vi "Mouse Left Click at Set Position.vi"(1 "Click position file path":path) -> (0 "Error out":errorcluster)   [LabVIEW 2015]
panel:
  out "Y":i32
  out "X":i32
  # "PN 18/11/2015"
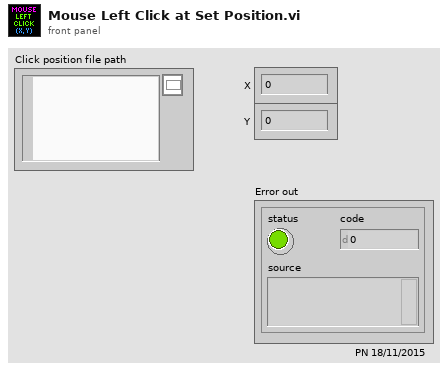
[diagram p1: front panel]
types:
  T1 = enum16{"open", "replace", "create", "open or create", "replace or create", "replace or create with confirmation"}
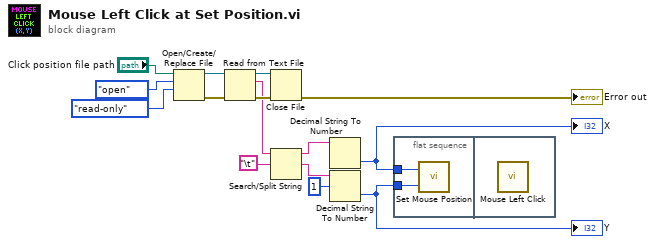
[diagram p0: block diagram]
diagram:
  n1 = Open/Create/Replace File(file path (use dialog)="Click position file path", operation (0:open)=T1."open", access (0:read/write)=enum16{"read/write", "read-only", "write-only"}."read-only") -> (refnum out=w14:refnum<file>, error out=w15:errorcluster)  [unwired: 3 in, 1 out]
  n2 = Read from Text File(file (use dialog)=w14, error in=w15) -> (refnum out=w10:refnum<file>, text=w4:string, error out=w9:errorcluster)  [unwired: 2 in, 1 out]
  n3 = Close File(refnum=w10, error in=w9) -> (error out=→"Error out":errorcluster)  [unwired: 1 out]
  n4 = Search/Split String(string=w4, search string/char (-)="\t") -> (substring before match=w2:string, match + rest of string=w1:string)  [unwired: 1 in, 1 out]
  n5 = Decimal String To Number(string=w2) -> (number=w7:i32)  [unwired: 2 in, 1 out]
  "X" <- w7
  n6 = Decimal String To Number(string=w1, offset=1) -> (number=w6:i32)  [unwired: 1 in, 1 out]
  "Y" <- w6
  n7 = flat-sequence {
    tunnel: w7 -> [w17]
    tunnel: w6 -> [w16]
    frame #0 {
      n8 = call "Set Mouse Position.vi"("Y"=w16, "X"=w17) -> ()  [unwired: 1 in]
    }
    frame #1 {
      n9 = call "Mouse Left Click.vi"() -> ()  [unwired: 1 in]
    }
  }
